vi "OpenAndUseFirstDevice.vi"(0 "object in":refnum<class "AD2_SDK.lvclass">, 5 "error in (no error)":errorcluster) -> (14 "object out":refnum<class "AD2_SDK.lvclass">, 19 "error out":errorcluster)   [LabVIEW 2019, in "AD2_SDK.lvclass"]
uses:
  AD2_SDK.lvclass
  AD2_SDK.lvclass/AD2_SDK.ctl
  Olasdwf/Olasdwf.lvlib
panel:
  out "function return":i32
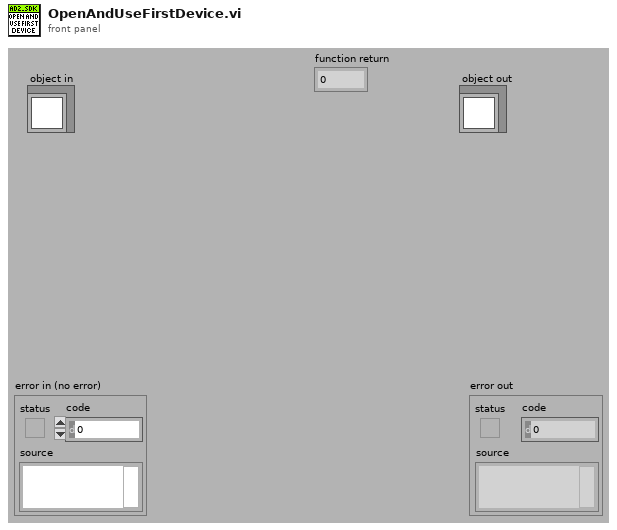
[diagram p1: front panel]
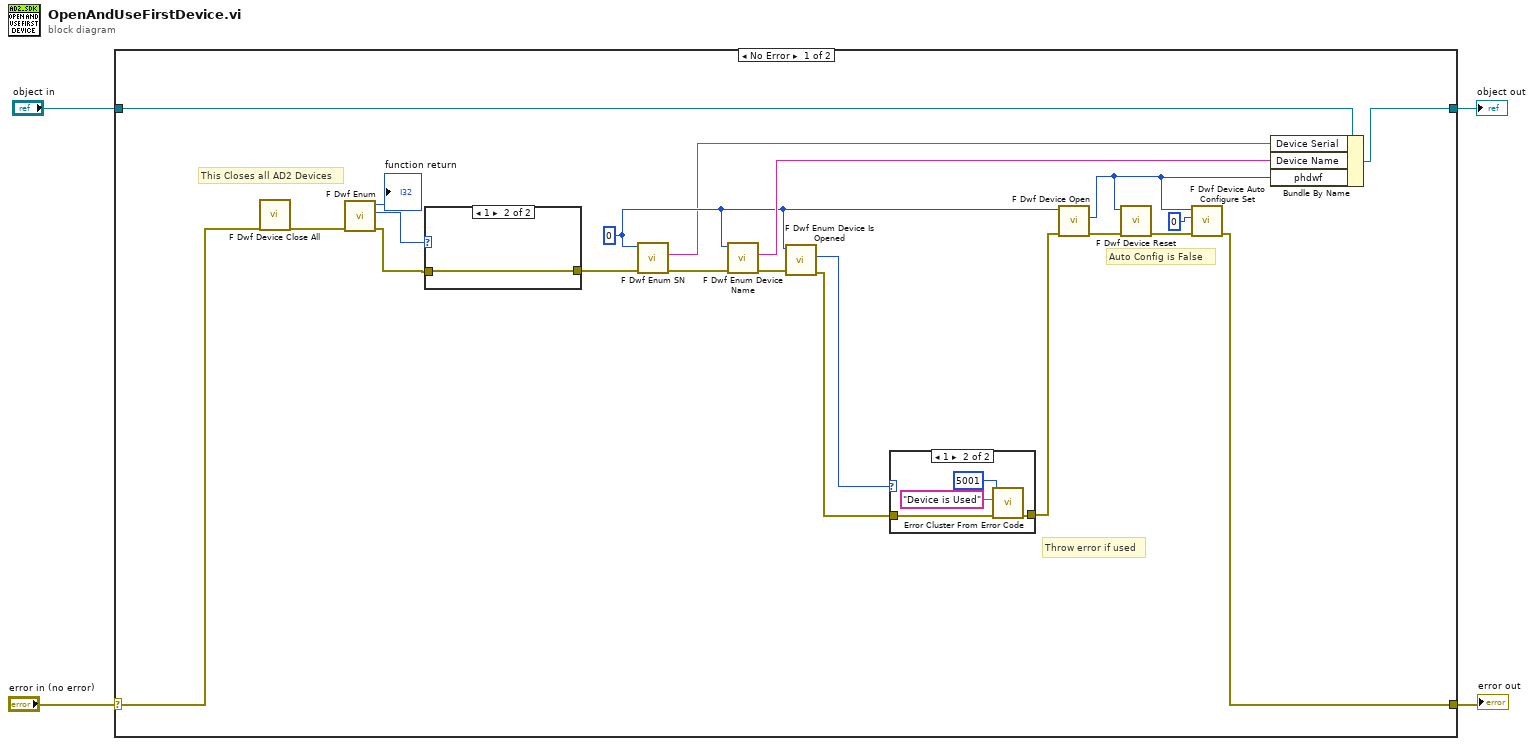
[diagram p0: block diagram]
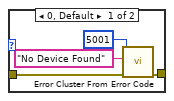
[diagram p2: hidden frame]
diagram:
  n1 = case shown="No Error" "error in (no error)" {
    selector: "error in (no error)" -> [w15 w37]
    tunnel: [w14 w37] -> w3
    tunnel: [w18 w36] -> w1
    tunnel: "object in" -> [w17 w36]
    frame No Error {
      w10 = 0 ("idxDevice")
      # "Auto Config is False"
      # "This Closes all AD2 Devices"
      # "Throw error if used"
      n2 = call "F Dwf Device Close All.vi"("error in (no error)"=w15) -> ("error out"=w23:errorcluster)  [unwired: 9 in, 1 out]
      n3 = call "F Dwf Enum.vi"("error in (no error)"=w23) -> ("error out"=w7:errorcluster, "pcDevice out"=w8:i32, "function return"=→"function return":i32)  [unwired: 8 in]
      n4 = case shown="1" w8 {
        tunnel: w7 -> [w28 w30]
        tunnel: [w27 w30] -> w6
        frame 0, Default {
          n5 = call <vilib>:"Error Cluster From Error Code.vi"("error in (no error)"=w28, "error message (\"\")"="No Device Found" ("error message (\"\")"), "error code (0)"=5001) -> ("error out"=w27:errorcluster)  [unwired: 6 in]
        }
        frame 1 {
        }
      }
      n6 = call "F Dwf Enum SN.vi"("error in (no error)"=w6, "idxDevice"=w10) -> ("error out"=w25:errorcluster, "szSN out"=w9:string)  [unwired: 7 in, 1 out]
      n7 = call "F Dwf Enum Device Name.vi"("error in (no error)"=w25, "idxDevice"=w10) -> ("error out"=w13:errorcluster, "szDeviceName out"=w24:string)  [unwired: 7 in, 1 out]
      n8 = call "F Dwf Enum Device Is Opened.vi"("error in (no error)"=w13, "idxDevice"=w10) -> ("error out"=w12:errorcluster, "pfIsUsed out"=w11:i32)  [unwired: 7 in, 1 out]
      n9 = case shown="1" w11 {
        tunnel: w12 -> [w31 w34]
        tunnel: [w31 w33] -> w16
        frame 0, Default {
        }
        frame 1 {
          n10 = call <vilib>:"Error Cluster From Error Code.vi"("error in (no error)"=w34, "error message (\"\")"="Device is Used" ("error message (\"\")"), "error code (0)"=5001) -> ("error out"=w33:errorcluster)  [unwired: 6 in]
        }
      }
      n11 = call "F Dwf Device Open.vi"("error in (no error)"=w16, "idxDevice"=w10) -> ("error out"=w22:errorcluster, "phdwf out"=w19:i32)  [unwired: 7 in, 1 out]
      n12 = call "F Dwf Device Reset.vi"("error in (no error)"=w22, "hdwf"=w19) -> ("error out"=w21:errorcluster)  [unwired: 8 in, 1 out]
      n13 = call "F Dwf Device Auto Configure Set.vi"("error in (no error)"=w21, "fAutoConfigure"=0, "hdwf"=w19) -> ("error out"=w14:errorcluster)  [unwired: 7 in, 1 out]
      n14 = Bundle By Name(cluster=w17, "Device Serial"=w9, "Device Name"=w24, "phdwf"=w19) -> (w18:refnum<class "AD2_SDK.lvclass">)
    }
    frame Error {
    }
  }
  "error out" <- w3
  "object out" <- w1
